vi "Write experimenter.vi"(8 "error in (no error)":errorcluster, 10 "experimenter":string, 11 "TimeStamper in":refnum<class "TimeStamper.lvclass">) -> (0 "error out":errorcluster, 3 "TimeStamper out":refnum<class "TimeStamper.lvclass">)   [LabVIEW 2014, in "TimeStamper.lvclass"]
uses:
  TimeStamper.lvclass
  TimeStamper.lvclass/TimeStamper.ctl
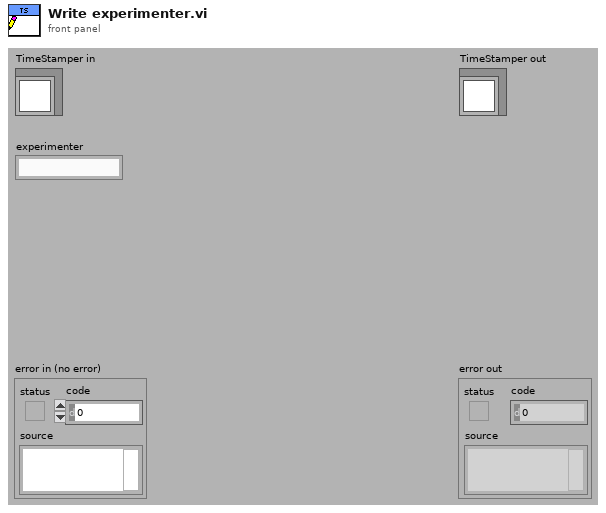
[diagram p1: front panel]
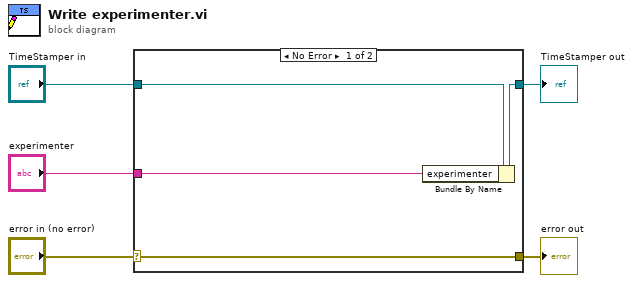
[diagram p0: block diagram]
diagram:
  n1 = case shown="No Error" "error in (no error)" {
    selector: "error in (no error)" -> [w9 w10]
    tunnel: [w9 w10] -> w4
    tunnel: [w7 w11] -> w2
    tunnel: "TimeStamper in" -> [w8 w11]
    tunnel: "experimenter" -> [w6 _]
    frame No Error {
      n2 = Bundle By Name(cluster=w8, "experimenter"=w6) -> (w7:refnum<class "TimeStamper.lvclass">)
    }
    frame Error {
    }
  }
  "error out" <- w4
  "TimeStamper out" <- w2
